vi "VectorToString.vi"(6 "format":string, 9 "vector length":i32, 10 "name":string, 11 "vector":dbl[](array[numeric])) -> (3 "string":string)   [LabVIEW 2011]
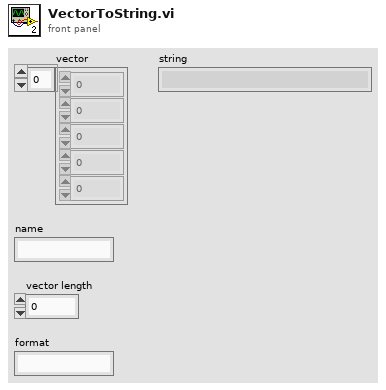
[diagram p1: front panel]
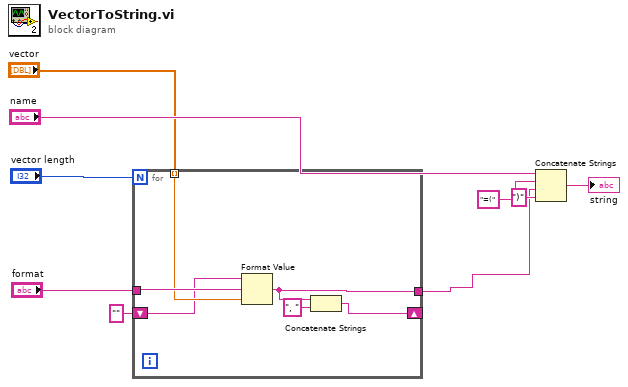
[diagram p0: block diagram]
diagram:
  n1 = for {
    N: "vector length" -> [_]
    tunnel: "vector" -> [w14] mode=indexing
    shift-right: [w11] -> _
    shift-left: "" -> [w13]
    tunnel: "format" -> [w15]
    tunnel: [w10] -> w7
    n2 = Format Value(string ("")=w13, format string=w15, value (0)=w14) -> (output string=w10:string)
    n3 = Concatenate Strings(w10, ", " ("string")) -> (w11:string)
  }
  n4 = Concatenate Strings("name", "=(" ("string"), w7, ")" ("string")) -> (→"string":string)
